vi "AI Read AFR.vi"(8 "Analog In":dbl[][](array[numeric]), 9 "Avg Point":i16[](array[numeric]), 10 "Intercept":dbl[](array[numeric]), 11 "Slope":dbl[](array[numeric])) -> (3 "Analog Out":T1)   [LabVIEW 2015]
uses:
  <vilib>/Analysis/baseanly.llb/Mean (DBL).vi
  <vilib>/Analysis/NI_AALBase.lvlib
  <vilib>/ptbypt/NI_PtbyPt.lvlib
panel:
  in  "Cluster":T1
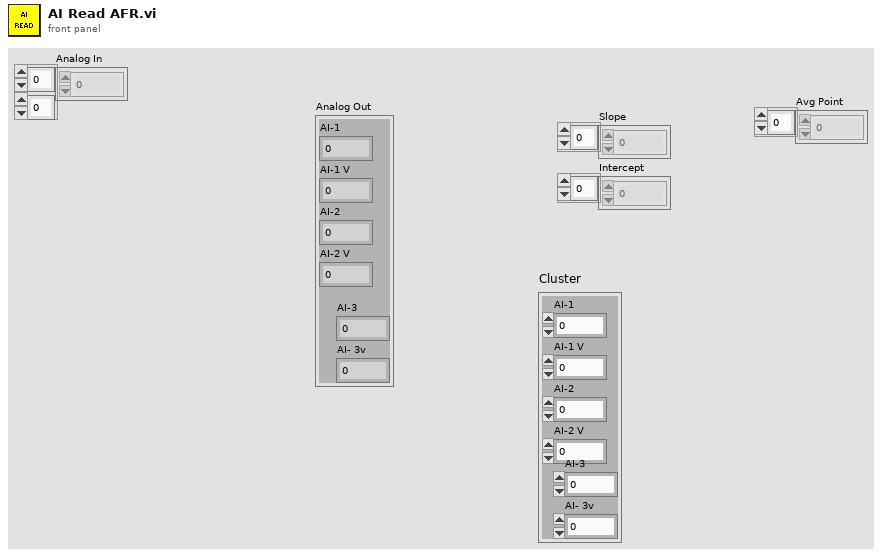
[diagram p1: front panel]
types:
  T1 = cluster{"AI-1":dbl, "AI-1 V":dbl, "AI-2":dbl, "AI-2 V":dbl, "AI-3":dbl, "AI- 3v":dbl}
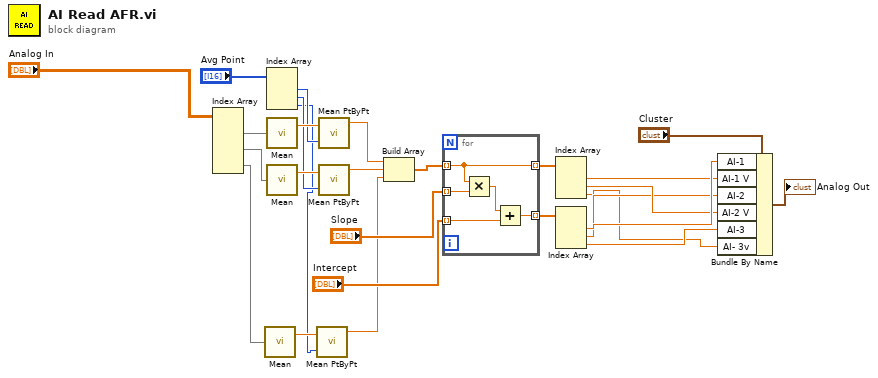
[diagram p0: block diagram]
diagram:
  n1 = Index Array(array="Analog In") -> (element #1=w10:dbl[], element #2=w9:dbl[], element #3=w6:dbl[])  [unwired: 6 in]
  n2 = call-poly <vilib>:"Mean.vi"("X"=w6) -> ("mean"=w5:dbl)  [unwired: 1 out]
  n3 = Index Array(array="Avg Point") -> (element #1=w25:i16, element #2=w24:i16, element #3=w4:i16)  [unwired: 3 in]
  n4 = call-poly <vilib>:"Mean.vi"("X"=w10) -> ("mean"=w27:dbl)  [unwired: 1 out]
  n5 = call-poly <vilib>:"Mean.vi"("X"=w9) -> ("mean"=w26:dbl)  [unwired: 1 out]
  n6 = call <vilib>:"Mean PtByPt.vi"("x"=w5, "sample length"=w4) -> ("mean"=w3:dbl)  [unwired: 2 in, 1 out]
  n7 = call <vilib>:"Mean PtByPt.vi"("x"=w27, "sample length"=w25) -> ("mean"=w19:dbl)  [unwired: 2 in, 1 out]
  n8 = call <vilib>:"Mean PtByPt.vi"("x"=w26, "sample length"=w24) -> ("mean"=w18:dbl)  [unwired: 2 in, 1 out]
  n9 = Build Array(w19, w18, w3) -> (w20:dbl[])
  n10 = for {
    tunnel: "Slope" -> [w32] mode=indexing
    tunnel: "Intercept" -> [w30] mode=indexing
    tunnel: w20 -> [w29] mode=indexing
    tunnel: [w29] -> w17 mode=indexing
    tunnel: [w28] -> w21 mode=indexing
    n11 = Multiply(x=w29, y=w32) -> (x*y=w31:dbl)
    n12 = Add(x=w31, y=w30) -> (x+y=w28:dbl)
  }
  n13 = Index Array(array=w17) -> (element #1=w14:dbl, element #2=w13:dbl, element #3=w1:dbl)  [unwired: 3 in]
  n14 = Index Array(array=w21) -> (element #1=w16:dbl, element #2=w11:dbl, element #3=w2:dbl)  [unwired: 3 in]
  n15 = Bundle By Name(cluster="Cluster", "AI-1"=w16, "AI-1 V"=w14, "AI-2"=w11, "AI-2 V"=w13, "AI-3"=w2, "AI- 3v"=w1) -> (→"Analog Out":T1)
